vi "Enriching Factory.vi"(5 "Slots":u32=3 min=3 max=9 step=2, 7 "Speed Upgrades":u32 max=8) -> (0 "Yellow Cake/s":ext, 1 "Uranium Ingots/s":ext, 2 "Yellow Cake/t":ext, 3 "Uranium Ingots/t":ext)   [LabVIEW 2023]
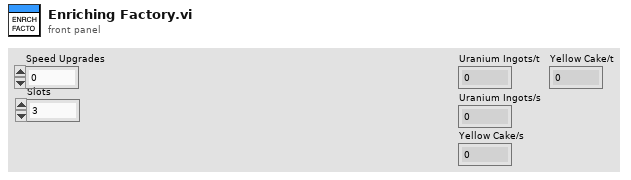
[diagram p1: front panel]
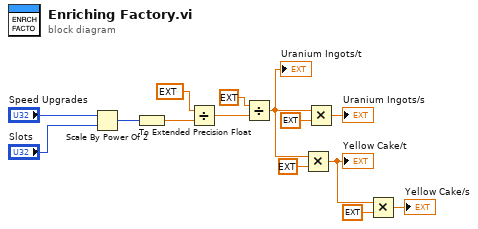
[diagram p0: block diagram]
diagram:
  n1 = Scale By Power Of 2(n="Speed Upgrades", x="Slots") -> (x*2^n=w2:u32)
  n2 = To Extended Precision Float(1:w2) -> (0:w1:ext)
  n3 = Divide(x=ext 200.0 ("y"), y=w1) -> (x/y=w10:ext)
  n4 = Divide(x=ext 1.0, y=w10) -> (x/y=w7:ext)
  "Uranium Ingots/t" <- w7
  n5 = Multiply(x=w7, y=ext 2.0) -> (x*y=w5:ext)
  "Yellow Cake/t" <- w5
  n6 = Multiply(x=w7, y=ext 20.0) -> (x*y=→"Uranium Ingots/s":ext)
  n7 = Multiply(x=w5, y=ext 20.0) -> (x*y=→"Yellow Cake/s":ext)
